vi "AIM Error Code to CD Error Code.vi"(8 "error in":errorcluster) -> (0 "error out":errorcluster, 1 "Numeric":i32, 2 "source minimum":string, 3 "source":string)   [LabVIEW 2020]
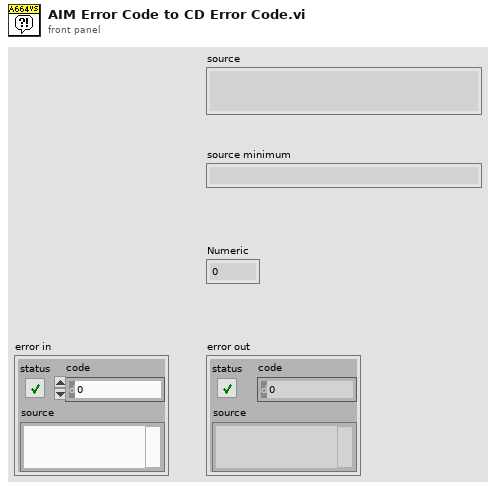
[diagram p1: front panel]
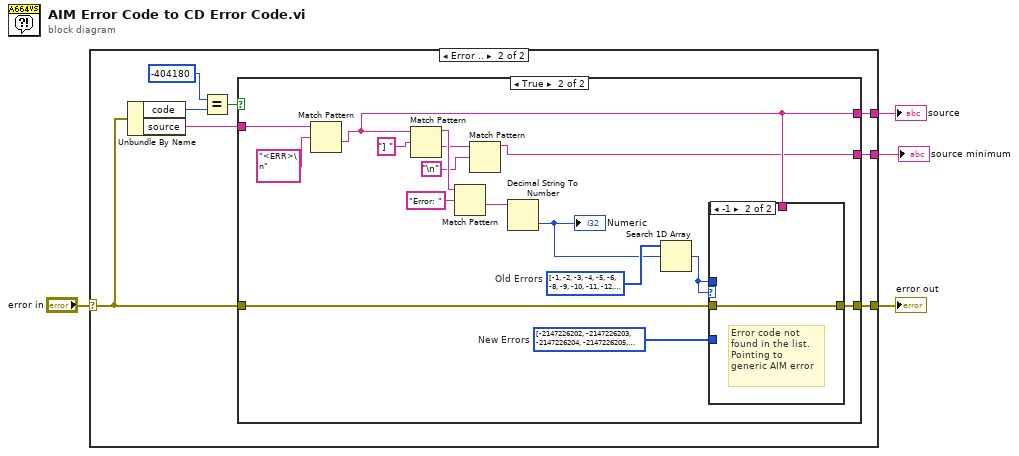
[diagram p0: block diagram]
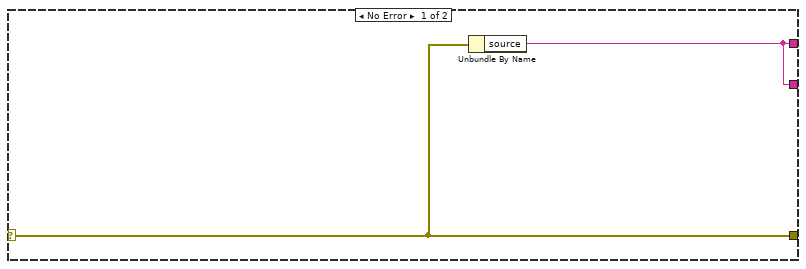
[diagram p2: hidden frame]
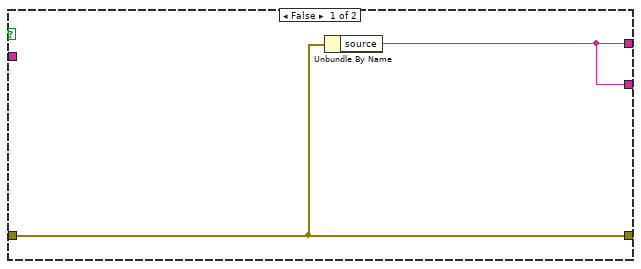
[diagram p3: hidden frame]
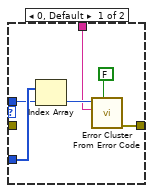
[diagram p4: hidden frame]
diagram:
  n1 = case shown="Error .." "error in" {
    selector: "error in" -> [w6 w9]
    tunnel: [w6 w13] -> w3
    tunnel: [w5 w10] -> w2
    tunnel: [w5 w7] -> w1
    frame No Error {
      n2 = Unbundle By Name(w6) -> ("source"=w5:string)
    }
    frame Error {
      n3 = Unbundle By Name(w9) -> ("code"=w12:i32, "source"=w14:string)
      n4 = Equal?(x=-404180 ("Numeric"), y=w12) -> (x = y?=w11:bool)
      n5 = case shown="True" w11 {
        tunnel: w14 -> [_ w28]
        tunnel: [w16 w21] -> w13
        tunnel: [w15 w20] -> w10
        tunnel: w9 -> [w16 w18]
        tunnel: [w15 w17] -> w7
        frame False {
          n6 = Unbundle By Name(w16) -> ("source"=w15:string)
        }
        frame True {
          w24 = i32[] [-1, -2, -3, -4, -5, -6, -8, -9, -10, -11, -12, -13, -14, -15, -16, -20, -900, -1000, -1001, -1212, -1213, -2001, -2002, -2003, -2100, -2101, -2102, -2103, -2104, -2110, -2120, -3001, -3002, -3003, -3004, -3005, -3006, -3007, -3008, -3009, -3010, -3011, -3012, -3013, -3380, -3381, -3382, -4000, -4001, -4002, -4003, -4004, -4005, -4006, -4007, -4008, -4009, -4010, -4011, -4012, -4100, -4200, -4201, -4202, -4203, -4204, -4205, -4206, -100000, -100001, -100002, -100003, -100004, -100005, -100006, -100007, -100008, -100009, -100010, -100011, -100012, -100013, -100014, -100015, -100016, -100017, -100018, -100019, -100020, -100021, -100022, -100023, -100024, -100025, -100026, -100027, -100028, -100029, -100030, -100031, -100032, -100033, -100034, -100035, -100036, -100037, -100038, -100039, -100040, -100041, -100042, -100043, -100044, -100045, -100046, -100047, -100048, -100049, -100050, -100051, -100052, -100053, -100054, -100055, -100056, -100057, -100058, -100059, -100060, -100061, -100062, -100063, -100064, -100065, -100066, -100067, -100068, -100069, -100070, -100071, -100072, -100073, -100074, -100075, -100076, -100077, -100078, -100079, -100080, -100081, -100082, -100083, -100084, -100085, -100086, -100087, -100088, -100089, -100090, -100091, -100092, -100093, -100094, -100095, -100096, -100097, -100098, -100099, -100100, -100101, -100102, -100103, -100104, -100105, -100106, -100107, -100108, -100109, -100110, -100111, -100112, -100113, -100114, -100115, -100116, -100117, -100118, -100119, -100120, -100121, -100122, -200000, -200001, -300001, -300002, -300003, -300004, -300005, -300006, -300007, -300008, -300009, -383614, -400051, -400099, -400100, -400101, -400102, -400104, -400105, -400106, -400107, -400108, -400111, -400150, -400201, -400202, -400203, -400204, -400301, -400302, -400303, -400304, -400305, -400306, -400307, -400308, -400309, -400311, -400312, -400313, -400314, -400315, -400317, -400318, -400319, -400320, -400321, -400322, -400331, -400332, -400333, -400340, -400351, -400353, -400360, -400361, -400362, -400363, -400364, -400365, -400366, -400370, -400371, -400372, -400373, -400377, -400380, -400381, -400382, -400383, -400384, -400385, -400400, -400401, -400402, -400403, -400404, -400405, -400406, -400407, -400409, -400456, -400457, -400458, -400500, -400501, -400502, -400503, -400504, -400505, -400550, -400551, -400552, -400553, -400554, -400555, -400600, -400601, -400604, -400605, -400606, -400608, -400610, -400620, -400650, -400651, -400653, -400654, -400655, -400656, -400658, -400659, -400660, -400670, -400671, -400700, -400701, -400710, -400711, -400780, -400781, -400782, -400784, -400790, -400820, -401001, -401002, -401003, -401101, -401102, -401103, -401104, -401201, -401202, -401203, -401208, -401211, -401212, -401306, -401307, -401308, -401309, -401311, -401312, -401313, -401317, -401318, -401321, -401322, -401323, -401400, -401502, -401601, -401603, -401604, -401605, -401611, -401612, -401613, -401614, -401701, -401702, -401703, -401801, -401802, -401803, -401901, -401910, -402000, -402001, -402002, -402003, -402004, -402005, -402006, -402007, -402008, -402009, -402020, -402021, -402022, -402023, -402024, -402025, -402026, -402027, -402028, -402029, -402030, -402031, -402032, -402033, -402034, -402035, -402036, -402037, -402038, -402039, -402040, -402041, -402051, -402052, -402053, -402054, -402055, -402061, -402062, -402063, -402064, -402100, -402101, -402102, -402103, -402104, -402105, -402106, -402107, -402108, -410000, -410001, -410002]  # Old Errors
          w22 = i32[] [-2147226202, -2147226203, -2147226204, -2147226205, -2147226206, -2147226207, -2147226208, -2147226209, -2147226210, -2147226211, -2147226212, -2147226213, -2147226214, -2147226215, -2147226216, -2147226217, -2147226218, -2147226219, -2147226220, -2147226221, -2147226222, -2147226223, -2147226224, -2147226225, -2147226226, -2147226227, -2147226228, -2147226229, -2147226230, -2147226231, -2147226232, -2147226233, -2147226234, -2147226235, -2147226236, -2147226237, -2147226238, -2147226239, -2147226240, -2147226241, -2147226242, -2147226243, -2147226244, -2147226245, -2147226246, -2147226247, -2147226248, -2147226249, -2147226250, -2147226251, -2147226252, -2147226253, -2147226254, -2147226255, -2147226256, -2147226257, -2147226258, -2147226259, -2147226260, -2147226261, -2147226262, -2147226263, -2147226264, -2147226265, -2147226266, -2147226267, -2147226268, -2147226269, -2147226270, -2147226271, -2147226272, -2147226273, -2147226274, -2147226275, -2147226276, -2147226277, -2147226278, -2147226279, -2147226280, -2147226281, -2147226282, -2147226283, -2147226284, -2147226285, -2147226286, -2147226287, -2147226288, -2147226289, -2147226290, -2147226291, -2147226292, -2147226293, -2147226294, -2147226295, -2147226296, -2147226297, -2147226298, -2147226299, -2147226300, -2147226301, -2147226302, -2147226303, -2147226304, -2147226305, -2147226306, -2147226307, -2147226308, -2147226309, -2147226310, -2147226311, -2147226312, -2147226313, -2147226314, -2147226315, -2147226316, -2147226317, -2147226318, -2147226319, -2147226320, -2147226321, -2147226322, -2147226323, -2147226324, -2147226325, -2147226326, -2147226327, -2147226328, -2147226329, -2147226330, -2147226331, -2147226332, -2147226333, -2147226334, -2147226335, -2147226336, -2147226337, -2147226338, -2147226339, -2147226340, -2147226341, -2147226342, -2147226343, -2147226344, -2147226345, -2147226346, -2147226347, -2147226348, -2147226349, -2147226350, -2147226351, -2147226352, -2147226353, -2147226354, -2147226355, -2147226356, -2147226357, -2147226358, -2147226359, -2147226360, -2147226361, -2147226362, -2147226363, -2147226364, -2147226365, -2147226366, -2147226367, -2147226368, -2147226369, -2147226370, -2147226371, -2147226372, -2147226373, -2147226374, -2147226375, -2147226376, -2147226377, -2147226378, -2147226379, -2147226380, -2147226381, -2147226382, -2147226383, -2147226384, -2147226385, -2147226386, -2147226387, -2147226388, -2147226389, -2147226390, -2147226391, -2147226392, -2147226393, -2147226394, -2147226395, -2147226396, -2147226397, -2147226398, -2147226399, -2147226400, -2147226401, -2147226402, -2147226403, -2147226404, -2147226405, -2147226406, -2147226407, -2147226408, -2147226409, -2147226410, -2147226411, -2147226412, -2147226413, -2147226414, -2147226415, -2147226416, -2147226417, -2147226418, -2147226419, -2147226420, -2147226421, -2147226422, -2147226423, -2147226424, -2147226425, -2147226426, -2147226427, -2147226428, -2147226429, -2147226430, -2147226431, -2147226432, -2147226433, -2147226434, -2147226435, -2147226436, -2147226437, -2147226438, -2147226439, -2147226440, -2147226441, -2147226442, -2147226443, -2147226444, -2147226445, -2147226446, -2147226447, -2147226448, -2147226449, -2147226450, -2147226451, -2147226452, -2147226453, -2147226454, -2147226455, -2147226456, -2147226457, -2147226458, -2147226459, -2147226460, -2147226461, -2147226462, -2147226463, -2147226464, -2147226465, -2147226466, -2147226467, -2147226468, -2147226469, -2147226470, -2147226471, -2147226472, -2147226473, -2147226474, -2147226475, -2147226476, -2147226477, -2147226478, -2147226479, -2147226480, -2147226481, -2147226482, -2147226483, -2147226484, -2147226485, -2147226486, -2147226487, -2147226488, -2147226489, -2147226490, -2147226491, -2147226492, -2147226493, -2147226494, -2147226495, -2147226496, -2147226497, -2147226498, -2147226499, -2147226500, -2147226501, -2147226502, -2147226503, -2147226504, -2147226505, -2147226506, -2147226507, -2147226508, -2147226509, -2147226510, -2147226511, -2147226512, -2147226513, -2147226514, -2147226515, -2147226516, -2147226517, -2147226518, -2147226519, -2147226520, -2147226521, -2147226522, -2147226523, -2147226524, -2147226525, -2147226526, -2147226527, -2147226528, -2147226529, -2147226530, -2147226531, -2147226532, -2147226533, -2147226534, -2147226535, -2147226536, -2147226537, -2147226538, -2147226539, -2147226540, -2147226541, -2147226542, -2147226543, -2147226544, -2147226545, -2147226546, -2147226547, -2147226548, -2147226549, -2147226550, -2147226551, -2147226552, -2147226553, -2147226554, -2147226555, -2147226556, -2147226557, -2147226558, -2147226559, -2147226560, -2147226561, -2147226562, -2147226563, -2147226564, -2147226565, -2147226566, -2147226567, -2147226568, -2147226569, -2147226570, -2147226571, -2147226572, -2147226573, -2147226574, -2147226575, -2147226576, -2147226577, -2147226578, -2147226579, -2147226580, -2147226581, -2147226582, -2147226583, -2147226584, -2147226585, -2147226586, -2147226587, -2147226588, -2147226589, -2147226590, -2147226591, -2147226592, -2147226593, -2147226594, -2147226595, -2147226596, -2147226597, -2147226598, -2147226599, -2147226600, -2147226601, -2147226602, -2147226603, -2147226604, -2147226605, -2147226606, -2147226607, -2147226608, -2147226609, -2147226610, -2147226611, -2147226612, -2147226613]  # New Errors
          n7 = Match Pattern(string=w28, regular expression="<ERR>\n") -> (after substring=w20:string)  [unwired: 1 in, 3 out]
          n8 = Match Pattern(string=w20, regular expression="] ") -> (before substring=w31:string, after substring=w29:string)  [unwired: 1 in, 2 out]
          n9 = Match Pattern(string=w31, regular expression="Error: ") -> (after substring=w32:string)  [unwired: 1 in, 3 out]
          n10 = Match Pattern(string=w29, regular expression="\n") -> (before substring=w17:string)  [unwired: 1 in, 3 out]
          n11 = Decimal String To Number(string=w32) -> (number=w23:i32)  [unwired: 2 in, 1 out]
          "Numeric" <- w23
          n12 = Search 1D Array(1D array=w24, element=w23) -> (index of element=w19:i32)  [unwired: 1 in]
          n13 = case shown="-1" w19 {
            tunnel: w22 -> [w38 _]
            tunnel: w19 -> [w37 _]
            tunnel: [w34 w39] -> w21
            tunnel: w20 -> [w33 _]
            tunnel: w18 -> [_ w39]
            frame 0, Default {
              n14 = Index Array(array=w38, index=w37) -> (element=w36:i32)
              n15 = call <vilib>:"Error Cluster From Error Code.vi"("show call chain? (False)"=FALSE, "error message (\"\")"=w33, "error code (0)"=w36) -> ("error out"=w34:errorcluster)  [unwired: 6 in]
            }
            frame -1 {
              # "Error code not \nfound in the list.\nPointing to \ngeneric AIM error"
            }
          }
        }
      }
    }
  }
  "error out" <- w3
  "source" <- w2
  "source minimum" <- w1
